vi "ConfigureIOMerge.vi"   [LabVIEW 2020]
doc: "Writes channel configuration data to the I/O items. Use this node with multiplexed analog input devices where the configuration for a channel transfers from the FPGA to the target I/O on each clock pulse. If the channel configuration does not update with each sample pulse, the previously written configuration transfers again, and the device will continue to acquire from the same channel with the same configuration."
uses:
  <vilib>/eio/EIOGrowableMethodNode/genericMethod/EIOGrowableMethodNode.xnode
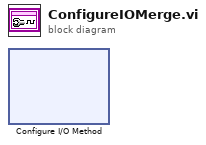
[diagram p0: block diagram]
diagram:
  n1 = xnode "Configure I/O Method"() -> ()  [unwired: 3 in, 2 out]
